vi "AWG Scale PreciseRamp Waveform amplitude for programming.vi"(8 "error in (no error)":errorcluster, 9 "AmpGain":i32, 10 "Waveform In":T1={"Start"=1.0, "End"=256.0, "Time"=1.0} caption="Cluster" {"Start" min=0.0 max=1.0 format="%.2f"; "Time" min=0.0 max=1.0 format="%.2f"}, 11 "Instrument Handle In":refnum<k15>) -> (0 "error out":errorcluster, 2 "Waveform Out":T1={"Start"=1.0, "End"=256.0, "Time"=1.0} caption="Waveform" {"Start" min=0.0 max=1.0 format="%.2f"; "Time" min=0.0 max=1.0 format="%.2f"}, 3 "Instrument Handle Out":refnum<k15>)   [LabVIEW 2013]
doc: "This VI reads the Gain and Offset of the AWG instrument and then rescales the amplitude of the waveform accordingly to range between -1 to 1 for programming the AWG instrument."
uses:
  PreciseRampWaveform.ctl
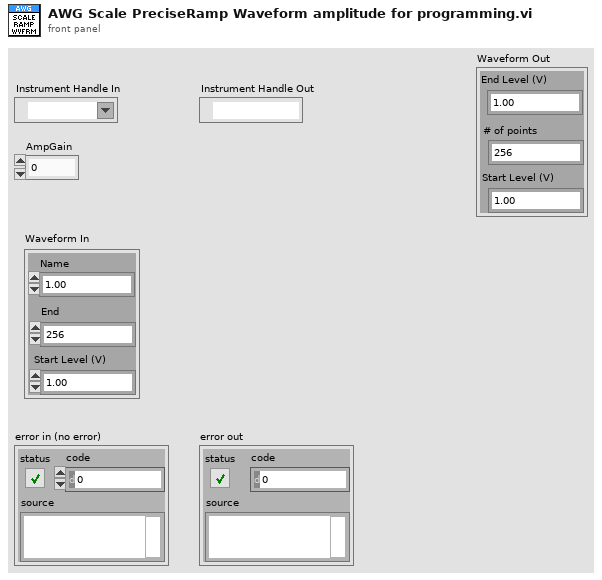
[diagram p1: front panel]
types:
  T1 = typedef "PreciseRampWaveform.ctl" = cluster{"Start":dbl, "End":dbl, "Time":dbl}
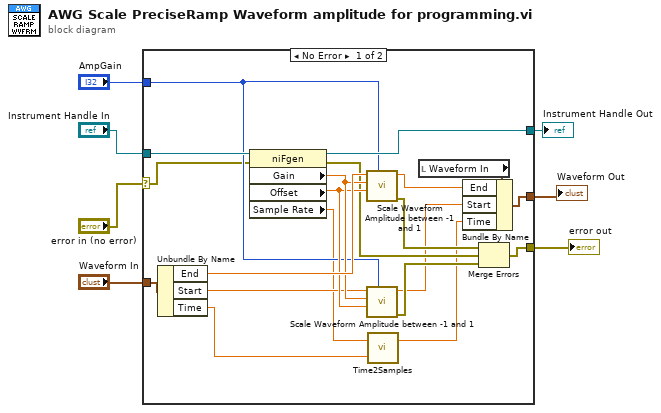
[diagram p0: block diagram]
diagram:
  n1 = case shown="No Error" "error in (no error)" {
    selector: "error in (no error)" -> [w11 w28]
    tunnel: [w27 _] -> w7
    tunnel: "Instrument Handle In" -> [w26 _]
    tunnel: [w25 w28] -> w5
    tunnel: "AmpGain" -> [w16 _]
    tunnel: [w13 _] -> w3
    tunnel: "Waveform In" -> [w12 _]
    frame No Error {
      n2 = Unbundle By Name(w12) -> ("End"=w23:dbl, "Start"=w15:dbl, "Time"=w9:dbl)
      n3 = property class="niFgen"(reference=w26, error in=w11) -> (reference out=w27:refnum<k15>, error out=w18:errorcluster, "Gain"=w20:dbl, "Offset"=w19:dbl, "Sample Rate"=w10:dbl)
      n4 = call "Scale Waveform Amplitude between -1 and 1.vi"("AmpGain"=w16, "Offset"=w19, "Gain"=w20, "Waveform Amplitude In (V)"=w23) -> ("error out"=w24:errorcluster, "Waveform Amplitude Out (-1 to 1)"=w21:dbl)  [unwired: 6 in]
      n5 = call "Scale Waveform Amplitude between -1 and 1.vi"("AmpGain"=w16, "Offset"=w19, "Gain"=w20, "Waveform Amplitude In (V)"=w15) -> ("error out"=w17:errorcluster, "Waveform Amplitude Out (-1 to 1)"=w14:dbl)  [unwired: 6 in]
      n6 = call "Time2Samples.vi"("Time"=w9, "SampleRate"=w10) -> ("Samples"=w8:dbl)  [unwired: 1 in]
      n7 = local read "Waveform In"() -> (w22:T1)
      n8 = Bundle By Name(cluster=w22, "End"=w21, "Start"=w14, "Time"=w8) -> (w13:T1)
      n9 = Merge Errors(w24, w18, w17) -> (w25:errorcluster)
    }
    frame Error {
    }
  }
  "error out" <- w5
  "Instrument Handle Out" <- w7
  "Waveform Out" <- w3
